vi "Run.vi"(8 "error in (no error)":errorcluster, 10 "Maze (0: Empty, -1: Enemy. >0: Teammate":i32[][](array[numeric]), 11 "Protect in":refnum<class "Protect.lvclass">) -> (0 "error out":errorcluster, 1 "Direction":T1, 2 "Action":T2, 3 "Protect out":refnum<class "Protect.lvclass">)   [LabVIEW 2014, in "Protect.lvclass"]
uses:
  Protect.lvclass
  Action Enum.ctl
  Direction Enum.ctl
  Maze 2.0.lvclass
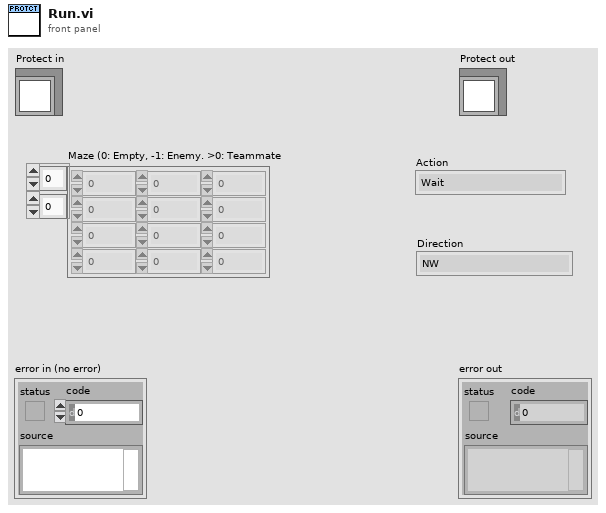
[diagram p1: front panel]
types:
  T1 = typedef "Maze 2.0.lvclass/Direction Enum.ctl" = enum16{"NW", "N", "NE", "E", "SE", "S", "SW", "W"}
  T2 = typedef "Maze 2.0.lvclass/Action Enum.ctl" = enum16{"Wait", "Move", "Attack", "Replicate"}
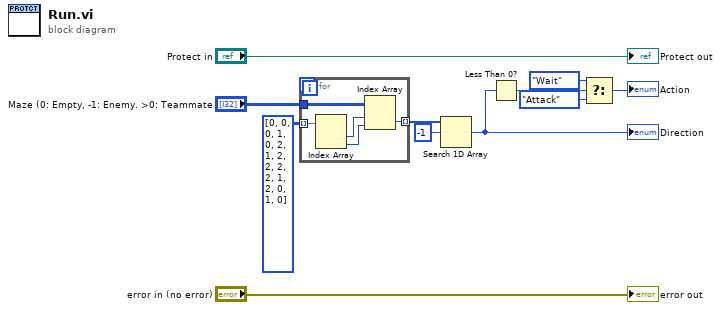
[diagram p0: block diagram]
diagram:
  n1 = for {
    tunnel: "Maze (0: Empty, -1: Enemy. >0: Teammate" -> [w16]
    tunnel: i32[][] [[0, 0], [0, 1], [0, 2], [1, 2], [2, 2], [2, 1], [2, 0], [1, 0]] -> [w15] mode=indexing
    tunnel: [w12] -> w6 mode=indexing
    n2 = Index Array(array=w15) -> (element #1=w14:i32, element #2=w13:i32)  [unwired: 2 in]
    n3 = Index Array(array=w16, index (row)=w14, index (col)=w13) -> (element=w12:i32)
  }
  n4 = Search 1D Array(1D array=w6, element=-1) -> (index of element=w5:i32)  [unwired: 1 in]
  "Direction" <- w5
  n5 = Less Than 0?(x=w5) -> (x < 0?=w4:bool)
  n6 = Select(t=Action_Enum."Wait" ("Action"), s=w4, f=Action_Enum."Attack" ("Action")) -> (s? t:f=→"Action":T2)
  "error out" <- "error in (no error)"
  "Protect out" <- "Protect in"
